vi "Ini_SetOutput.vi"(8 "error in (no error)":errorcluster, 11 "ZanCard in":refnum<class "ZanCard.lvclass">) -> (0 "error out":errorcluster, 3 "ZanCard out":refnum<class "ZanCard.lvclass">)   [LabVIEW 2019, in "ZanCard.lvclass"]
uses:
  ZanCard.lvclass
  ZanCard.lvclass/ZanCard.ctl
  LLB/zmotion/zaux/zauxdll.lvlib
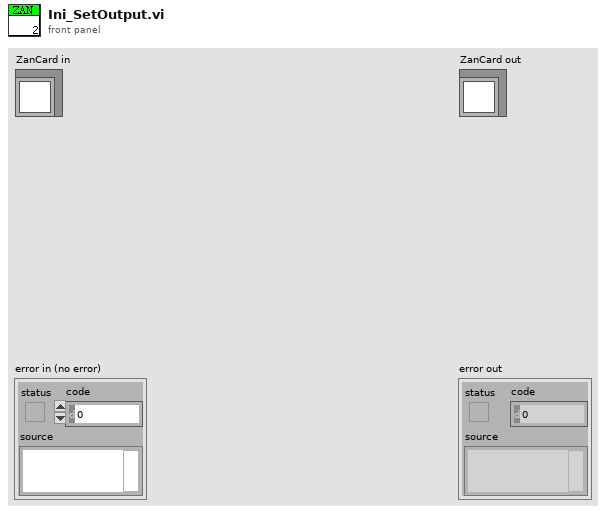
[diagram p1: front panel]
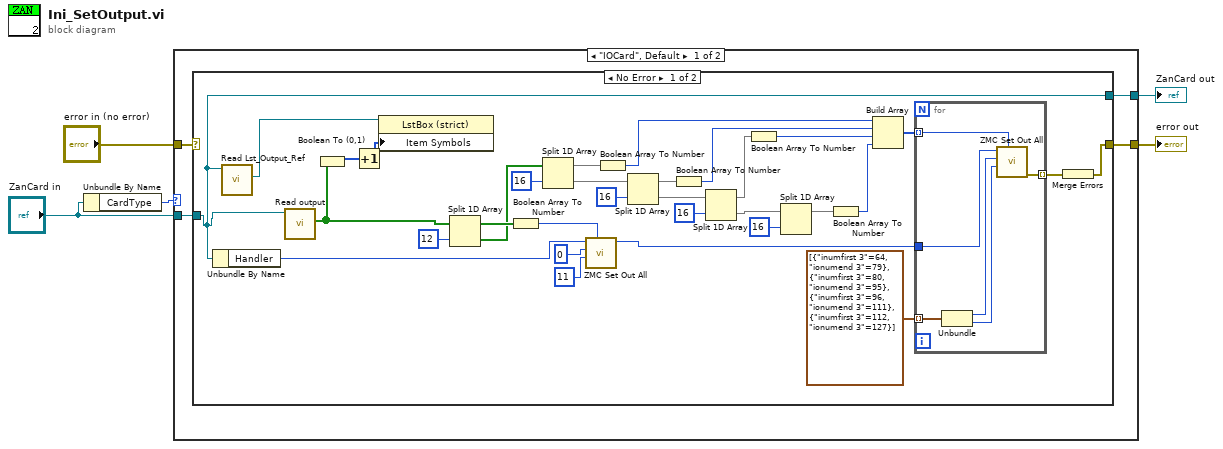
[diagram p0: block diagram]
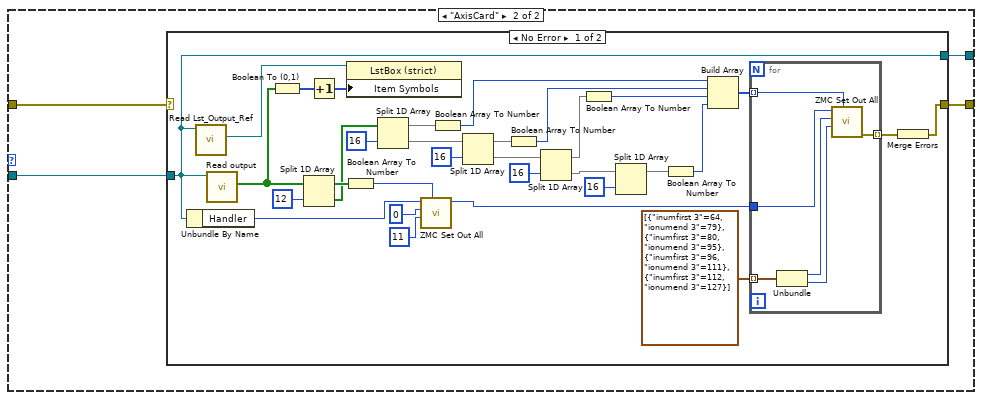
[diagram p3: hidden frame]
diagram:
  n1 = Unbundle By Name("ZanCard in") -> ("CardType"=w1:enum16{"AxisCard", "IOCard"})
  n2 = case shown="\"IOCard\", Default" w1 {
    tunnel: [w9 w53] -> w5
    tunnel: [w8 w52] -> w4
    tunnel: "ZanCard in" -> [w7 w51]
    tunnel: "error in (no error)" -> [w6 w50]
    frame "IOCard", Default {
      n3 = case shown="No Error" w6 {
        selector: w6 -> [_ w48]
        tunnel: w7 -> [w13 w49]
        tunnel: [w14 w48] -> w9
        tunnel: [w13 w49] -> w8
        frame No Error {
          n4 = Unbundle By Name(w13) -> ("Handler"=w35:i32)
          n5 = call-dynamic "Read Lst_Output_Ref.vi"("IOCard in"=w13) -> ("Lst_Output_Ref"=w38:refnum<vi>)  [unwired: 8 in, 2 out]
          n6 = call-dynamic "Read output.vi"("IOCard in"=w13) -> ("output"=w12:bool[])  [unwired: 8 in, 2 out]
          n7 = Boolean To (0,1)(Boolean=w12) -> (0, 1=w11:i16[])
          n8 = Increment(x=w11) -> (x+1=w10:i16[])
          n9 = property class="LstBox (strict)"(reference=w38, "Item Symbols"=w10) -> ()  [unwired: 1 in, 2 out]
          n10 = Split 1D Array(array=w12, index=12) -> (first subarray=w36:bool[], second subarray=w34:bool[])
          n11 = Boolean Array To Number(Boolean array=w36) -> (number=w39:u32)
          n12 = Split 1D Array(array=w34, index=16) -> (first subarray=w30:bool[], second subarray=w31:bool[])
          n13 = call "ZMC Set Out All.vi"("istate"=w39, "inumend"=u16 11, "inumfirst"=u16 0 ("inumend"), "handle"=w35) -> ("handle out"=w17:u32)  [unwired: 5 in, 2 out]
          n14 = Boolean Array To Number(Boolean array=w30) -> (number=w22:u32)
          n15 = Split 1D Array(array=w31, index=16) -> (first subarray=w29:bool[], second subarray=w26:bool[])
          n16 = Boolean Array To Number(Boolean array=w29) -> (number=w21:u32)
          n17 = Split 1D Array(array=w26, index=16) -> (first subarray=w28:bool[], second subarray=w23:bool[])
          n18 = Boolean Array To Number(Boolean array=w28) -> (number=w20:u32)
          n19 = Split 1D Array(array=w23, index=16) -> (first subarray=w24:bool[])  [unwired: 1 out]
          n20 = Boolean Array To Number(Boolean array=w24) -> (number=w19:u32)
          n21 = Build Array(w22, w21, w20, w19) -> (w18:u32[])
          n22 = for {
            tunnel: w18 -> [w47] mode=indexing
            tunnel: w17 -> [w46]
            tunnel: cluster{"inumfirst 3":u16, "ionumend 3":i32}[] [{"inumfirst 3"=64, "ionumend 3"=79}, {"inumfirst 3"=80, "ionumend 3"=95}, {"inumfirst 3"=96, "ionumend 3"=111}, {"inumfirst 3"=112, "ionumend 3"=127}] -> [w45] mode=indexing
            tunnel: [w42] -> w15 mode=indexing
            n23 = Unbundle(w45) -> ("inumfirst 3"=w44:u16, "ionumend 3"=w43:i32)
            n24 = call "ZMC Set Out All.vi"("istate"=w47, "inumend"=w43, "inumfirst"=w44, "handle"=w46) -> ("error out"=w42:errorcluster)  [unwired: 5 in, 2 out]
          }
          n25 = Merge Errors(w15) -> (w14:errorcluster)
        }
        frame Error {
        }
      }
    }
    frame "AxisCard" {
      n26 = case shown="No Error" w50 {
        selector: w50 -> [_ w92]
        tunnel: w51 -> [w82 w93]
        tunnel: [w54 w92] -> w53
        tunnel: [w82 w93] -> w52
        frame No Error {
          n27 = Unbundle By Name(w82) -> ("Handler"=w75:i32)
          n28 = call-dynamic "Read Lst_Output_Ref.vi"("IOCard in"=w82) -> ("Lst_Output_Ref"=w81:refnum<vi>)  [unwired: 8 in, 2 out]
          n29 = call-dynamic "Read output.vi"("IOCard in"=w82) -> ("output"=w77:bool[])  [unwired: 8 in, 2 out]
          n30 = Boolean To (0,1)(Boolean=w77) -> (0, 1=w80:i16[])
          n31 = Split 1D Array(array=w77, index=12) -> (first subarray=w76:bool[], second subarray=w74:bool[])
          n32 = Increment(x=w80) -> (x+1=w79:i16[])
          n33 = Boolean Array To Number(Boolean array=w76) -> (number=w83:u32)
          n34 = property class="LstBox (strict)"(reference=w81, "Item Symbols"=w79) -> ()  [unwired: 1 in, 2 out]
          n35 = Split 1D Array(array=w74, index=16) -> (first subarray=w70:bool[], second subarray=w71:bool[])
          n36 = call "ZMC Set Out All.vi"("istate"=w83, "inumend"=u16 11, "inumfirst"=u16 0 ("inumend"), "handle"=w75) -> ("handle out"=w57:u32)  [unwired: 5 in, 2 out]
          n37 = Boolean Array To Number(Boolean array=w70) -> (number=w62:u32)
          n38 = Split 1D Array(array=w71, index=16) -> (first subarray=w69:bool[], second subarray=w66:bool[])
          n39 = Boolean Array To Number(Boolean array=w69) -> (number=w61:u32)
          n40 = Split 1D Array(array=w66, index=16) -> (first subarray=w68:bool[], second subarray=w63:bool[])
          n41 = Boolean Array To Number(Boolean array=w68) -> (number=w60:u32)
          n42 = Split 1D Array(array=w63, index=16) -> (first subarray=w64:bool[])  [unwired: 1 out]
          n43 = Boolean Array To Number(Boolean array=w64) -> (number=w59:u32)
          n44 = Build Array(w62, w61, w60, w59) -> (w58:u32[])
          n45 = for {
            tunnel: w58 -> [w91] mode=indexing
            tunnel: w57 -> [w90]
            tunnel: cluster{"inumfirst 3":u16, "ionumend 3":i32}[] [{"inumfirst 3"=64, "ionumend 3"=79}, {"inumfirst 3"=80, "ionumend 3"=95}, {"inumfirst 3"=96, "ionumend 3"=111}, {"inumfirst 3"=112, "ionumend 3"=127}] -> [w89] mode=indexing
            tunnel: [w86] -> w55 mode=indexing
            n46 = Unbundle(w89) -> ("inumfirst 3"=w88:u16, "ionumend 3"=w87:i32)
            n47 = call "ZMC Set Out All.vi"("istate"=w91, "inumend"=w87, "inumfirst"=w88, "handle"=w90) -> ("error out"=w86:errorcluster)  [unwired: 5 in, 2 out]
          }
          n48 = Merge Errors(w55) -> (w54:errorcluster)
        }
        frame Error {
        }
      }
    }
  }
  "error out" <- w5
  "ZanCard out" <- w4
